vi "Launch Preview Actor.vi"(8 "error in (no error)":errorcluster, 11 "Cfg Grandmaster in":refnum<class "Cfg Grandmaster.lvclass">) -> (0 "error out":errorcluster, 3 "Cfg Grandmaster out":refnum<class "Cfg Grandmaster.lvclass">)   [LabVIEW 2012, in "Configuration Grandmaster.lvlib" / "Cfg Grandmaster.lvclass"]
uses:
  Cfg Grandmaster.lvclass
  Cfg Grandmaster.lvclass/Cfg Grandmaster.ctl
  <vilib>/ActorFramework/Actor/Actor.lvclass/Actor.ctl
  <vilib>/ActorFramework/Message Enqueuer/Message Enqueuer.lvclass/Message Enqueuer.ctl
  <vilib>/ActorFramework/Message Enqueuer/Init from Existing Queue.vi
  <vilib>/ActorFramework/Message Enqueuer/Message Enqueuer.lvclass
  Preview Window/Class Preview/Preview.lvclass
  Actor Nest/Class Actor Nest/Actor Nest.lvclass
  <vilib>/ActorFramework/Actor/Actor.lvclass
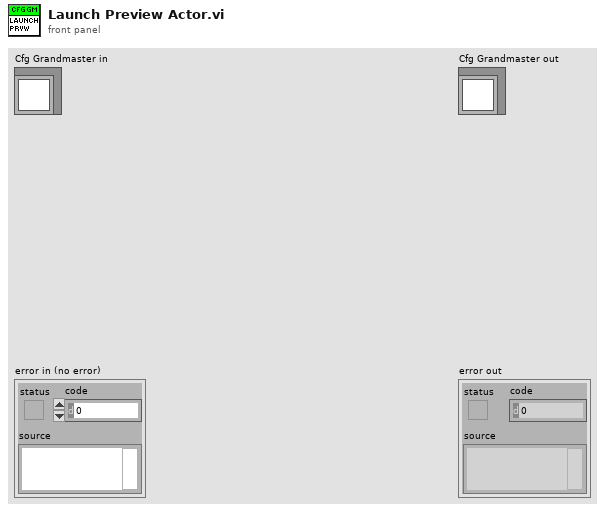
[diagram p1: front panel]
types:
  T1 = typedef "ge_Cfg wChassis.ctl" = cluster{"Chassis BOM":refnum<class "Chassis BOM.lvclass">, "Chassis Cfg":refnum<class "ChassisCfg.lvclass">, "Chassis Tasks":refnum<class "Chassis Tasks.lvclass">, "HW Error":bool, "Unsvd Chgs?":bool}
  T2 = typedef "Selected Group.ctl" = cluster{"ChanGroup":i32, "Rate Class":T3}
  T3 = typedef "TE_Designator.ctl" = enum16{"High Speed", "Low Speed"}
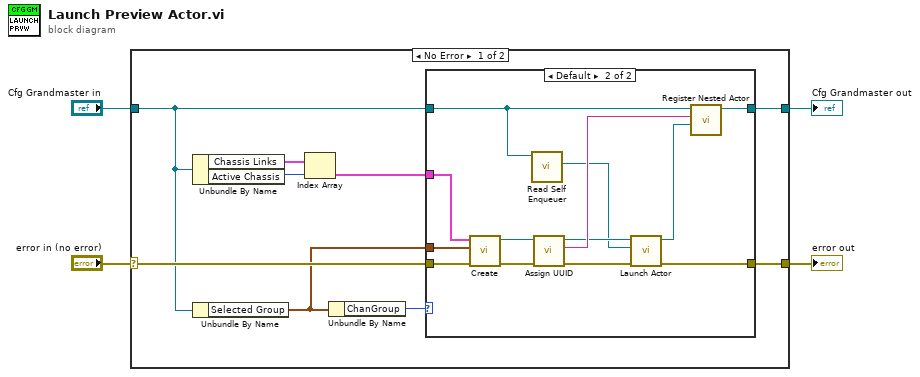
[diagram p0: block diagram]
diagram:
  n1 = case shown="No Error" "error in (no error)" {
    selector: "error in (no error)" -> [w11 w30]
    tunnel: [w12 w30] -> w3
    tunnel: [w5 w29] -> w1
    tunnel: "Cfg Grandmaster in" -> [w9 w29]
    frame No Error {
      n2 = Unbundle By Name(w9) -> ("Chassis Links"=w8:T1[], "Active Chassis"=w7:i32)
      n3 = Unbundle By Name(w9) -> ("Selected Group"=w10:T2)
      n4 = Index Array(array=w8, index=w7) -> (element=w6:T1)
      n5 = Unbundle By Name(w10) -> ("ChanGroup"=w13:i32)
      n6 = case shown="Default" w13 {
        tunnel: [w14 w18] -> w12
        tunnel: w9 -> [w15 w17]
        tunnel: w11 -> [w14 w26]
        tunnel: w10 -> [_ w25]
        tunnel: w6 -> [_ w24]
        tunnel: [w15 w19] -> w5
        frame -1 {
        }
        frame Default {
          n7 = call "Create.vi"("error in (no error)"=w26, "Selected Group"=w25, "Chassis Link"=w24) -> ("error out"=w27:errorcluster, "Preview out"=w28:refnum<class "Preview.lvclass">)  [unwired: 7 in]
          n8 = call <vilib>:"Read Self Enqueuer.vi"("Actor"=w17) -> ("Self Enqueuer"=w16:refnum<class "Message Enqueuer.lvclass">)  [unwired: 10 in]
          n9 = call "Assign UUID.vi"("error in (no error)"=w27, "Actor Nest in"=w28) -> ("error out"=w21:errorcluster, "String UUID"=w23:string, "Actor Nest out"=w22:refnum<class "Preview.lvclass">)  [unwired: 7 in]
          n10 = call <vilib>:"Launch Actor.vi"("error in (no error)"=w21, "Actor-to-Caller Enqueuer"=w16, "Actor"=w22) -> ("error out"=w18:errorcluster, "Caller-To-Actor Enqueuer"=w20:refnum<class "Message Enqueuer.lvclass">)  [unwired: 7 in]
          n11 = call-dynamic "Register Nested Actor.vi"("Caller-To-Actor Enqueuer"=w20, "Actor UUID"=w23, "Actor Nest in"=w17) -> ("Actor Nest out"=w19:refnum<class "Cfg Grandmaster.lvclass">)  [unwired: 7 in, 1 out]
        }
      }
    }
    frame Error {
    }
  }
  "error out" <- w3
  "Cfg Grandmaster out" <- w1
